vi "NI-USB6525.vi"() -> ()   [LabVIEW 2020]
doc: "test"
uses:
  LabVIEW 2020 Toolkits/toolkits_lv2020_32bit/Synchronization.llb/SynchRefs_SetGet.ctl
  LabVIEW 2020 Toolkits/VI Server Toolkit/VI Server Libraries/VI Server_GetControl.llb/VI Server_STR_Get.vi
  LabVIEW 2020 Toolkits/VI Server Toolkit/VI Server Libraries/VI Server_Set Controls.llb/Set STR Control.vi
  LabVIEW 2020 Toolkits/VI Server Toolkit/VI Server Libraries/VI Server_SetControl.llb/VI Server_BOOL_Set.vi
  LabVIEW 2020 Toolkits/VI Server Toolkit/VI Server Libraries/VI Server_SetControl.llb/VI Server_U32_Set.vi
  LabVIEW 2020 Toolkits/VI Server Toolkit/VI Server Libraries/VI Server_SetControl.llb/VI Server_1D_BOOL_Set.vi
  LabVIEW 2020 Toolkits/VI Server Toolkit/VI Server Libraries/VI Server_GetControl.llb/VI Server_DAQmx_Device_Get.vi
  LabVIEW 2020 Toolkits/VI Server Toolkit/VI Server Toolkit LV2013.lvlib
panel:
  in  "LastAction.AddToSecuence":bool
  in  "Help":bool
  in  "FP.Hide":bool caption="FrontPanel.Hide"
  out "System.Message":string caption="System Message"
  in  "EXIT":bool
  in  "Tab.Main":enum32{"Digital I/O", "Sequence", "SETTINGS"}(tab)
  in  "DataConverter.Number":u8 caption="Number"
  in  "DataConverter.Array":bool[](array[boolean])
  out "DI.Number":u8 caption="DI Number"
  out "Relay.State.Verify":bool caption="Verified"
  in  "RelayPort.Num":u8
  in  "Relay.RST":bool
  in  "RelayPort":bool[](array[boolean]) caption="Relay Port"
  out "Relay.Port.State.Verify":bool caption="Verified"
  in  "R8":bool
  in  "R7":bool
  in  "R6":bool
  in  "R5":bool
  in  "R4":bool
  in  "R3":bool
  in  "R2":bool
  in  "R1":bool
  out "DI.8":bool caption="DI 8"
  out "DI.7":bool caption="DI 7"
  out "DI.6":bool caption="DI 6"
  out "DI.5":bool caption="DI 5"
  out "DI.4":bool caption="DI 4"
  out "DI.3":bool caption="DI 3"
  out "DI.2":bool caption="DI 2"
  out "DI.1":bool caption="DI 1"
  in  "TestCase.Execute.All":bool
  in  "TestCase.Execute.Selected":bool
  out "TestCase.SAVE.Success":bool
  in  "TestCase.SAVE":bool
  in  "SequenceFile.Open":bool
  in  "SequenceFile":path caption="Secuence File"
  in  "TestCase.Execute.Step.Pause":bool
  in  "TestCase.Execute.Steps":u16(ring) caption="Test Case: Pause Before Step" items=["1", "2", "3", "4", "5", "6", "7", "8", "9", "10", "11", "12", "13", "14", "15", "16", "17", "18", "19", "20", "21", "22", "23", "24", "25", "26", "27", "28", "29", "30"]
  in  "TestCase.Execute.ABORT":bool
  in  "TestCase.Execute.Next":bool
  in  "TestCase.Execute.Pause":bool
  out "TestCase.ExecutionTime":dbl caption="Execution Time:" format="%0.3f sec"
  in  "TestCase.Execution.StepTime":u32 caption="Seq. Execution: Step Time" format="%d msec"
  in  "TestCaseConfiguration":i32[](listbox) caption="Test Case Configuration"
  in  "TestCase.StepDescription":string caption="Step Description:"
  in  "UDP.Test.String1.SendLocal":bool caption="UDP.Test.String1.Send"
  in  "ProductType":string="NI-USB6525" caption="Product Type"
  in  "VI.WindowsTitle":string="NI-USB6525" caption="Windows Title"
  in  "DAQmx.Device":tag="NI-USB6525" caption="DAQmx: Device"
  in  "Cont.Measurements.CycleTime":u32 caption="Continius Measurements:\nCycleTime"
  in  "UDP.Test.String2.Send":bool
  in  "UDP.Test.String2":string caption="UDP: Test String 2"
  in  "UDP.Port.BC":u16=58433 caption="UDP: Port.BC"
  in  "UDP.Port.RT":u16=58432 caption="UDP: Port.RT"
  in  "UDP.LocalPort":u16=58434 caption="UDP: Local Port"
  in  "UDP.IP.Address":string="234.5.6.7" caption="UDP: IP Address"
  in  "UDP.Test.String1.Send.ToInstr":bool caption="UDP.Test.String1.Send"
  in  "UDP.Test.String1":string caption="UDP: Test String 1"
  in  "UDP.Responce.String.Monitor":bool
  out "UDP.ExecEng.Message.String":string caption="UDP: Execution Engine Message String"
  out "error out":errorcluster={"status"=TRUE, "code"=1055, "source"="Property Node in VI Server Toolkit LV2013.lvlib:VI server_Set Control Value from String Format.vi:5200001->DMM6500_UDP_ExecEng_Instruction_APPLY.vi->DMM6500_UDP_MAIN.vi->Keithley2100.vi"}
  in  "error in":errorcluster
  # "15JUN2022"
  # "Digital Inputs"
  # "Data Converter"
  # "RELAYS"
  # "ON"
  # "OFF"
  # "M"
  # "Multicast IP addresses must be in the 224.0.0.0 to 239.255.255.255 range."
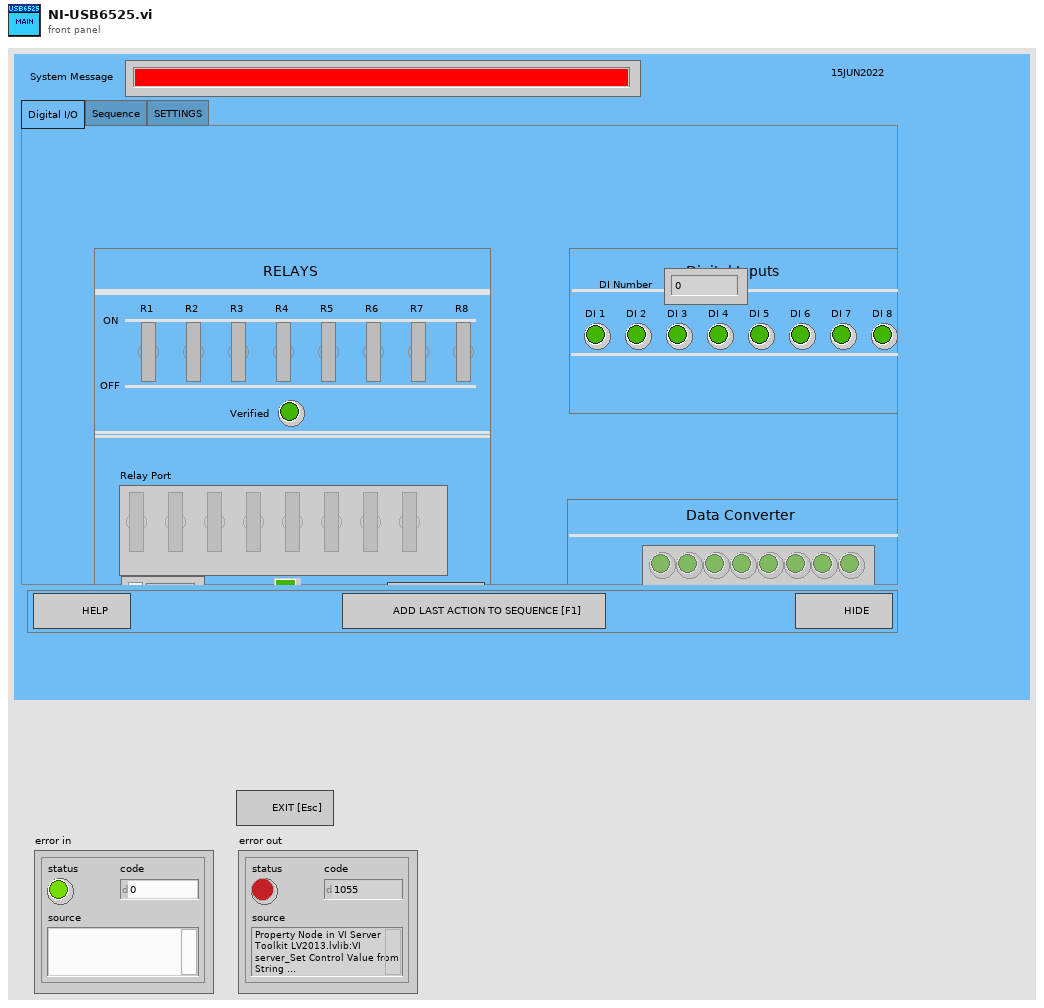
[diagram p1: front panel]
types:
  T1 = typedef "VI Server_RefsCluster.ctl" = cluster{"Labels":string[], "Refs":refnum<vi>[], "VI Ref":refnum<vi>}
  T2 = typedef "SynchRefs_SetGet.ctl" = enum16{"Set", "Get"}
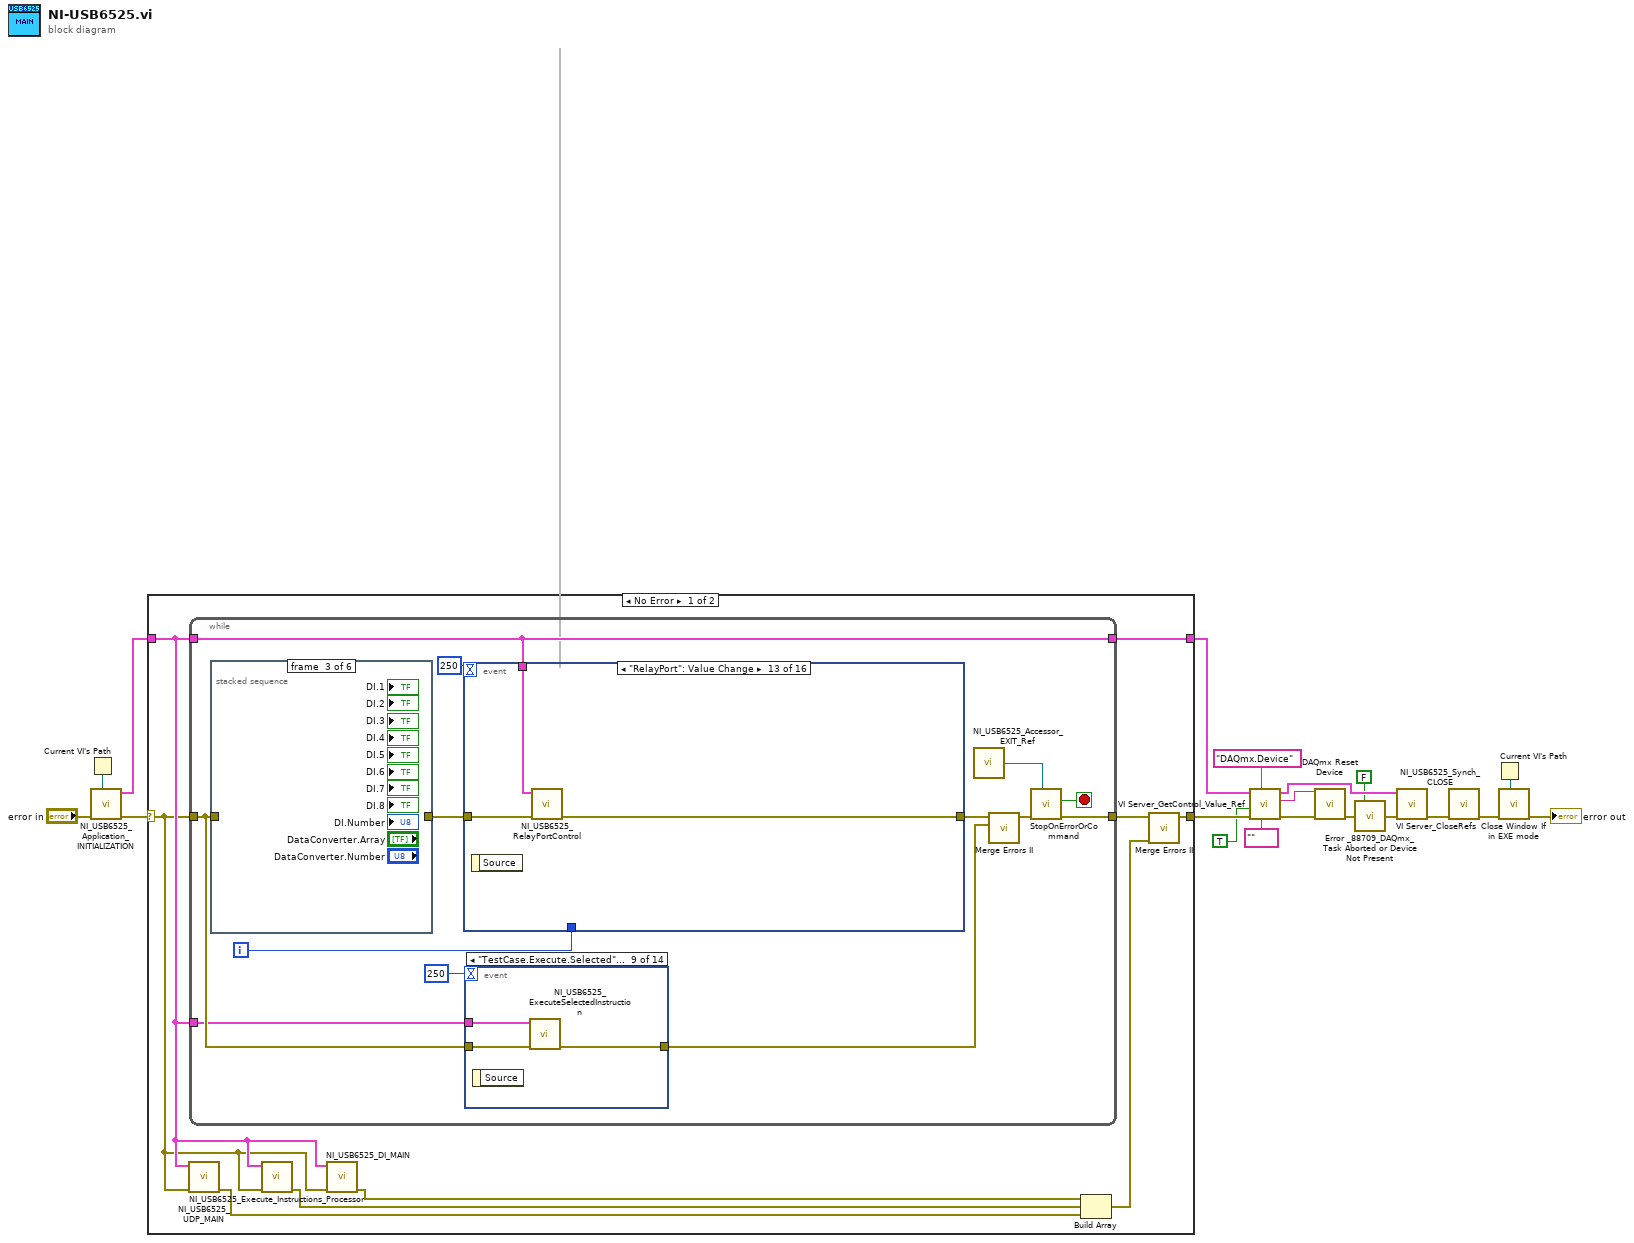
[diagram p0: block diagram]
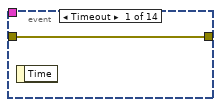
[diagram p2: hidden frame]
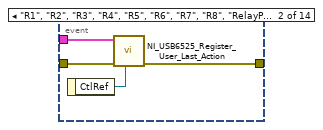
[diagram p3: hidden frame]
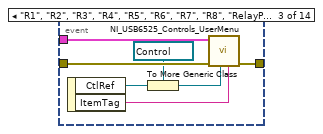
[diagram p4: hidden frame]
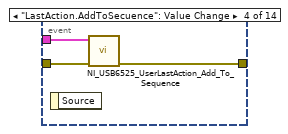
[diagram p5: hidden frame]
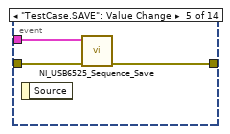
[diagram p6: hidden frame]
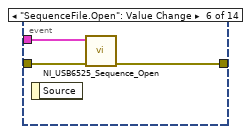
[diagram p7: hidden frame]
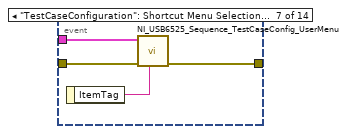
[diagram p8: hidden frame]
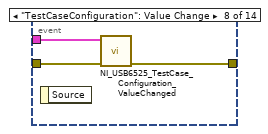
[diagram p9: hidden frame]
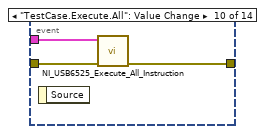
[diagram p10: hidden frame]
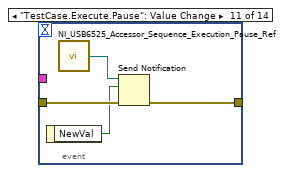
[diagram p11: hidden frame]
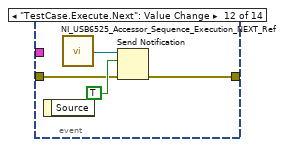
[diagram p12: hidden frame]
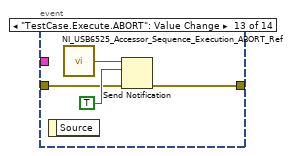
[diagram p13: hidden frame]
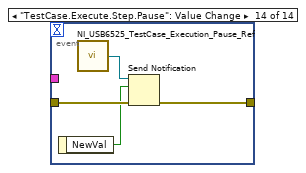
[diagram p14: hidden frame]
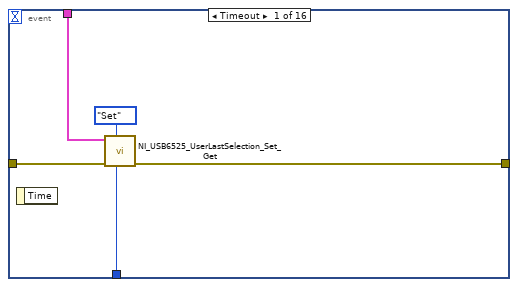
[diagram p15: hidden frame]
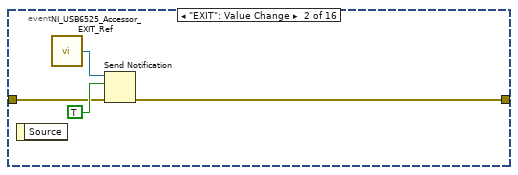
[diagram p16: hidden frame]
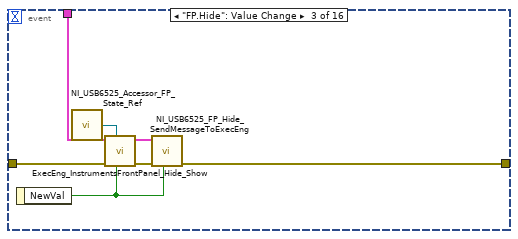
[diagram p17: hidden frame]
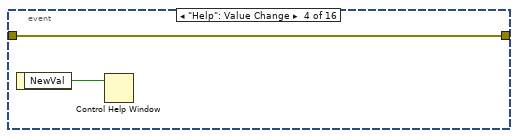
[diagram p18: hidden frame]
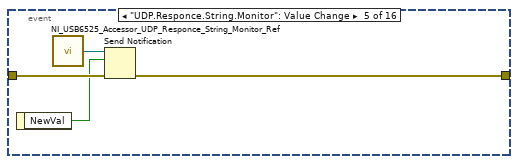
[diagram p19: hidden frame]
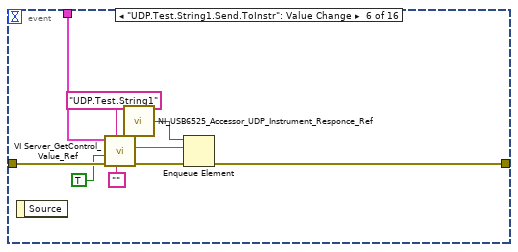
[diagram p20: hidden frame]
diagram:
  n1 = Current VI's Path() -> (path=w3:path)
  n2 = call "NI_USB6525_Application_INITIALIZATION.vi"("Top VI Path"=w3, "error in (no error)"="error in") -> ("error out"=w19:errorcluster, "VI Server Cluster.OUT"=w2:T1)  [unwired: 8 in]
  n3 = case shown="No Error" w19 {
    selector: w19 -> [w21 w192]
    tunnel: [w25 w192] -> w13
    tunnel: w2 -> [w22 w191]
    tunnel: [w28 w191] -> w11
    frame No Error {
      n4 = call "NI_USB6525_UDP_MAIN.vi"("error in (no error)"=w21, "VI Server.RefsCluster"=w22) -> ("error out"=w27:errorcluster)  [unwired: 9 in]
      n5 = while {
        tunnel: w21 -> [w33]
        tunnel: [w37] -> w26
        tunnel: w22 -> [w38]
        tunnel: [w38] -> w28
        tunnel: w22 -> [w29]
        i -> [w39]
        stop <- w36 stop-if-true
        n6 = stacked-sequence {
          tunnel: w33 -> [w190 _ _ _ _ _]
          tunnel: [w190 _ _ _ _ _] -> w41
          frame #0 {
          }
          frame #1 {
          }
          frame #2 {
          }
          frame #3 {
          }
          frame #4 {
          }
          frame #5 {
          }
        }
        n7 = event shown="[12] \"RelayPort\": Value Change" {
          selector: _ -> [_ _ _ _ _ _ _ _ _ _ _ _ _ _ _ _]
          dyn-events: _ -> [_ _ _ _ _ _ _ _ _ _ _ _ _ _ _ _]
          timeout: 250 -> [_ _ _ _ _ _ _ _ _ _ _ _ _ _ _ _]
          tunnel: w41 -> [w95 w97 w107 w109 w113 w122 w131 w140 w144 w155 w158 w168 w172 w175 w181 w188]
          tunnel: w39 -> [w94 _ _ _ _ _ _ _ _ _ _ _ _ _ _ _]
          tunnel: [w92 w99 w102 w109 w111 w120 w129 w138 w142 w153 w161 w169 w171 w173 w176 w187] -> w32
          tunnel: w38 -> [w93 _ w106 _ _ w119 w128 w137 w141 w154 w156 w166 w170 w174 w178 w186]
          event Timeout {
            n8 = event-data() -> ()  [unwired: 1 in, 1 out]
            n9 = call "NI_USB6525_UserLastSelection_Set_Get.vi"("LoopCounter"=w94, "SynchRefs.Set/Get"=SynchRefs_SetGet."Set", "error in"=w95, "VI Server.RefsCluster"=w93) -> ("error out"=w92:errorcluster)  [unwired: 6 in, 1 out]
          }
          event "EXIT": Value Change {
            n10 = event-data() -> ()  [unwired: 1 in, 1 out]
            n11 = call "NI_USB6525_Accessor_EXIT_Ref.vi"() -> ("EXIT"=w100:refnum<notifier>)  [unwired: 6 in]
            n12 = Send Notification(notification=TRUE, notifier=w100, error in (no error)=w97) -> (error out=w99:errorcluster)  [unwired: 1 out]
          }
          event "FP.Hide": Value Change {
            n13 = event-data() -> ("NewVal"=w101:bool)  [unwired: 1 in]
            n14 = call "NI_USB6525_Accessor_FP_State_Ref.vi"() -> ("FP.State"=w105:refnum<notifier>)  [unwired: 6 in]
            n15 = call "ExecEng_InstrumentsFrontPanel_Hide_Show.vi"("FP.Hide/Show"=w101, "FP.State"=w105, "error in (no error)"=w107, "VI Server Cluster"=w106) -> ("error out"=w103:errorcluster, "VI Server Cluster DUP"=w104:T1)  [unwired: 6 in]
            n16 = call "NI_USB6525_FP_Hide_SendMessageToExecEng.vi"("FP.Open"=w101, "error in (no error)"=w103, "VI Server Cluster"=w104) -> ("error out"=w102:errorcluster)  [unwired: 8 in]
          }
          event "Help": Value Change {
            n17 = event-data() -> ("NewVal"=w108:bool)  [unwired: 1 in]
            n18 = Control Help Window(1:w108) -> ()  [unwired: 1 in]
          }
          event "UDP.Responce.String.Monitor": Value Change {
            n19 = event-data() -> ("NewVal"=w110:bool)  [unwired: 1 in]
            n20 = call "NI_USB6525_Accessor_UDP_Responce_String_Monitor_Ref.vi"() -> ("UDP.ExecEng.Command.String.Monitor"=w112:refnum<notifier>)  [unwired: 6 in]
            n21 = Send Notification(notification=w110, notifier=w112, error in (no error)=w113) -> (error out=w111:errorcluster)  [unwired: 1 out]
          }
          event "UDP.Test.String1.Send.ToInstr": Value Change {
            n22 = event-data() -> ()  [unwired: 1 in, 1 out]
            n23 = call-poly "VI Server_GetControl_Value_Ref.vi"("DataType"="", "Control.Label"="UDP.Test.String1", "error in"=w122, "SingleInstance"=TRUE, "VI Server.RefsCluster"=w119) -> ("error out"=w121:errorcluster, "Value"=w114:string)  [unwired: 3 in, 2 out]
            n24 = call "NI_USB6525_Accessor_UDP_Instrument_Responce_Ref.vi"() -> ("UDP.Instrument.Responce.Q"=w115:refnum<queue>)  [unwired: 6 in]
            n25 = Enqueue Element(queue=w115, element=w114, error in (no error)=w121) -> (error out=w120:errorcluster)  [unwired: 1 in, 2 out]
          }
          event "UDP.Test.String1.SendLocal": Value Change {
            n26 = event-data() -> ()  [unwired: 1 in, 1 out]
            n27 = call-poly "VI Server_GetControl_Value_Ref.vi"("DataType"="", "Control.Label"="UDP.Test.String1", "error in"=w131, "SingleInstance"=TRUE, "VI Server.RefsCluster"=w128) -> ("error out"=w130:errorcluster, "Value"=w124:string)  [unwired: 3 in, 2 out]
            n28 = call "NI_USB6525_Accessor_UDP_ExecEng_Instruction_Q_Ref.vi"() -> ("UDP.ExecEng.Instruction.Q"=w123:refnum<queue>)  [unwired: 6 in]
            n29 = Enqueue Element(queue=w123, element=w124, error in (no error)=w130) -> (error out=w129:errorcluster)  [unwired: 1 in, 2 out]
          }
          event "UDP.Test.String2.Send": Value Change {
            n30 = event-data() -> ()  [unwired: 1 in, 1 out]
            n31 = call-poly "VI Server_GetControl_Value_Ref.vi"("DataType"="", "Control.Label"="UDP.Test.String2", "error in"=w140, "SingleInstance"=TRUE, "VI Server.RefsCluster"=w137) -> ("error out"=w139:errorcluster, "Value"=w132:string)  [unwired: 3 in, 2 out]
            n32 = call "NI_USB6525_Accessor_UDP_Instrument_Responce_Ref.vi"() -> ("UDP.Instrument.Responce.Q"=w133:refnum<queue>)  [unwired: 6 in]
            n33 = Enqueue Element(queue=w133, element=w132, error in (no error)=w139) -> (error out=w138:errorcluster)  [unwired: 1 in, 2 out]
          }
          event "UDP.ExecEng.Message.String": Shortcut Menu Selection (User) {
            n34 = event-data() -> ("ItemTag"=w143:string)  [unwired: 1 in]
            n35 = case shown="\"Clear Indicator\"" w143 {
              tunnel: w144 -> [w145 w151]
              tunnel: [w145 w150] -> w142
              tunnel: w141 -> [_ w149]
              frame "", Default {
              }
              frame "Clear Indicator" {
                n36 = call-poly "VI Server_Set Control Value.vi"("New Value"="", "Label"="UDP.ExecEng.Message.String" ("Control.Label"), "error in"=w151, "Single Instance (T)"=TRUE ("SingleInstance"), "VI Server Cluster"=w149) -> ("error out"=w150:errorcluster)  [unwired: 4 in, 2 out]
              }
            }
          }
          event "DAQmx.Device": Value Change {
            n37 = event-data() -> ("NewVal"=w152:tag)  [unwired: 1 in]
            n38 = call "NI_USB6525_DAQmx_DeviceName_Changed_UpdateSet_Get_Sections.vi"("DAQmx.Device"=w152, "error in (no error)"=w155, "VI Server Cluster"=w154) -> ("error out"=w153:errorcluster)  [unwired: 8 in]
          }
          event "Relay.RST": Value Change {
            n39 = event-data() -> ()  [unwired: 1 in, 1 out]
            n40 = call "NI_USB6525_Relays_RST.vi"("error in (no error)"=w158, "VI Server Cluster"=w156) -> ("error out"=w159:errorcluster, "VI Server Cluster.DUP"=w157:T1)  [unwired: 8 in]
            n41 = call "Time Delay"("error in (no error)"=w159, "Delay Time (s)"=0.75) -> ("error out"=w164:errorcluster)  [unwired: 9 in]
            n42 = call-poly "VI Server_SetControl.vi"("Data"=FALSE ("SingleInstance"), "Control.Label"="Relay.RST", "error in"=w164, "SingleInstance"=TRUE, "VI Server.RefsCluster"=w157) -> ("error out"=w161:errorcluster)  [unwired: 4 in, 2 out]
          }
          event "R1", "R2", "R3", "R4", "R5", "R6", "R7", "R8": Value Change {
            n43 = event-data() -> ("CtlRef"=w167:refnum<vi>)  [unwired: 1 in]
            n44 = call "NI_USB6525_RelayControl.vi"("Relay.Ref"=w167, "error in (no error)"=w168, "VI Server Cluster"=w166) -> ("error out"=w169:errorcluster)  [unwired: 8 in]
          }
          event "RelayPort": Value Change {
            n45 = event-data() -> ()  [unwired: 1 in, 1 out]
            n46 = call "NI_USB6525_RelayPortControl.vi"("error in (no error)"=w172, "VI Server Cluster"=w170) -> ("error out"=w171:errorcluster)  [unwired: 9 in]
          }
          event "RelayPort.Num": Value Change {
            n47 = event-data() -> ()  [unwired: 1 in, 1 out]
            n48 = call "NI_USB6525_RelayPortControl_Numeric.vi"("error in (no error)"=w175, "VI Server Cluster"=w174) -> ("error out"=w173:errorcluster)  [unwired: 9 in]
          }
          event "DataConverter.Array": Value Change {
            n49 = event-data() -> ("NewVal"=w182:bool[])  [unwired: 1 in]
            n50 = Boolean Array To Number(Boolean array=w182) -> (number=w179:u32)
            n51 = call-poly "VI Server_SetControl.vi"("Data"=w179, "Control.Label"="DataConverter.Number", "error in"=w181, "SingleInstance"=TRUE, "VI Server.RefsCluster"=w178) -> ("error out"=w176:errorcluster)  [unwired: 4 in, 2 out]
          }
          event "DataConverter.Number": Value Change {
            n52 = event-data() -> ("NewVal"=w189:u8)  [unwired: 1 in]
            n53 = Number To Boolean Array(number=w189) -> (Boolean array=w185:bool[])
            n54 = call-poly "VI Server_SetControl.vi"("Data"=w185, "Control.Label"="DataConverter.Array", "error in"=w188, "SingleInstance"=TRUE, "VI Server.RefsCluster"=w186) -> ("error out"=w187:errorcluster)  [unwired: 5 in, 1 out]
          }
        }
        n55 = event shown="[8] \"TestCase.Execute.Selected\": Value Change" {
          selector: _ -> [_ _ _ _ _ _ _ _ _ _ _ _ _ _]
          dyn-events: _ -> [_ _ _ _ _ _ _ _ _ _ _ _ _ _]
          timeout: 250 -> [_ _ _ _ _ _ _ _ _ _ _ _ _ _]
          tunnel: w33 -> [w42 w46 w52 w56 w59 w62 w66 w69 w72 w75 w78 w81 w85 w90]
          tunnel: [w42 w44 w51 w55 w57 w60 w63 w67 w70 w73 w77 w80 w84 w89] -> w30
          tunnel: w29 -> [_ w45 w53 w54 w58 w61 w65 w68 w71 w74 _ _ _ _]
          event Timeout {
            n56 = event-data() -> ()  [unwired: 1 in, 1 out]
          }
          event "R1", "R2", "R3", "R4", "R5", "R6", "R7", "R8", "RelayPort", "Relay.RST", "RelayPort.Num": Value Change {
            n57 = event-data() -> ("CtlRef"=w43:refnum<vi>)  [unwired: 1 in]
            n58 = call "NI_USB6525_Register_User_Last_Action.vi"("CtlRef"=w43, "error in (no error)"=w46, "VI Server Cluster"=w45) -> ("error out"=w44:errorcluster)  [unwired: 7 in, 1 out]
          }
          event "R1", "R2", "R3", "R4", "R5", "R6", "R7", "R8", "RelayPort.Num", "Relay.RST", "RelayPort": Shortcut Menu Selection (User) {
            n59 = event-data() -> ("CtlRef"=w48:refnum<vi>, "ItemTag"=w50:string)  [unwired: 1 in]
            n60 = To More Generic Class(target class=refnum<vi> refnum ("Control Reference (Generic)"), reference=w48) -> (generic class reference=w47:refnum<vi>)
            n61 = call "NI_USB6525_Controls_UserMenu.vi"("ItemTag"=w50, "Control Ref"=w47, "error in (no error)"=w52, "VI Server Cluster"=w53) -> ("error out"=w51:errorcluster)  [unwired: 7 in]
          }
          event "LastAction.AddToSecuence": Value Change {
            n62 = event-data() -> ()  [unwired: 1 in, 1 out]
            n63 = call "NI_USB6525_UserLastAction_Add_To_Sequence.vi"("error in (no error)"=w56, "VI Server Cluster"=w54) -> ("error out"=w55:errorcluster)  [unwired: 9 in]
          }
          event "TestCase.SAVE": Value Change {
            n64 = event-data() -> ()  [unwired: 1 in, 1 out]
            n65 = call "NI_USB6525_Sequence_Save.vi"("error in (no error)"=w59, "VI Server Cluster"=w58) -> ("error out"=w57:errorcluster)  [unwired: 9 in]
          }
          event "SequenceFile.Open": Value Change {
            n66 = event-data() -> ()  [unwired: 1 in, 1 out]
            n67 = call "NI_USB6525_Sequence_Open.vi"("error in (no error)"=w62, "VI Server Cluster"=w61) -> ("error out"=w60:errorcluster)  [unwired: 9 in]
          }
          event "TestCaseConfiguration": Shortcut Menu Selection (User) {
            n68 = event-data() -> ("ItemTag"=w64:string)  [unwired: 1 in]
            n69 = call "NI_USB6525_Sequence_TestCaseConfig_UserMenu.vi"("ItemTag"=w64, "error in (no error)"=w66, "VI Server.RefsCluster"=w65) -> ("error out"=w63:errorcluster)  [unwired: 8 in]
          }
          event "TestCaseConfiguration": Value Change {
            n70 = event-data() -> ()  [unwired: 1 in, 1 out]
            n71 = call "NI_USB6525_TestCase_Configuration_ValueChanged.vi"("error in"=w69, "VI Server.RefsCluster"=w68) -> ("error out"=w67:errorcluster)  [unwired: 8 in, 1 out]
          }
          event "TestCase.Execute.Selected": Value Change {
            n72 = event-data() -> ()  [unwired: 1 in, 1 out]
            n73 = call "NI_USB6525_ExecuteSelectedInstruction.vi"("error in (no error)"=w72, "VI Server Cluster"=w71) -> ("error out"=w70:errorcluster)  [unwired: 9 in]
          }
          event "TestCase.Execute.All": Value Change {
            n74 = event-data() -> ()  [unwired: 1 in, 1 out]
            n75 = call "NI_USB6525_Execute_All_Instruction.vi"("error in (no error)"=w75, "VI Server Cluster"=w74) -> ("error out"=w73:errorcluster)  [unwired: 9 in]
          }
          event "TestCase.Execute.Pause": Value Change {
            n76 = event-data() -> ("NewVal"=w76:bool)  [unwired: 1 in]
            n77 = call "NI_USB6525_Accessor_Sequence_Execution_Pause_Ref.vi"() -> ("SequenceExecution.PAUSE"=w79:refnum<notifier>)  [unwired: 6 in]
            n78 = Send Notification(notification=w76, notifier=w79, error in (no error)=w78) -> (error out=w77:errorcluster)  [unwired: 1 out]
          }
          event "TestCase.Execute.Next": Value Change {
            n79 = event-data() -> ()  [unwired: 1 in, 1 out]
            n80 = call "NI_USB6525_Accessor_Sequence_Execution_NEXT_Ref.vi"() -> ("SequenceExecution.NEXT"=w83:refnum<notifier>)  [unwired: 6 in]
            n81 = Send Notification(notification=TRUE, notifier=w83, error in (no error)=w81) -> (error out=w80:errorcluster)  [unwired: 1 out]
          }
          event "TestCase.Execute.ABORT": Value Change {
            n82 = event-data() -> ()  [unwired: 1 in, 1 out]
            n83 = call "NI_USB6525_Accessor_Sequence_Execution_ABORT_Ref.vi"() -> ("SequenceExecution.ABORT"=w86:refnum<notifier>)  [unwired: 6 in]
            n84 = Send Notification(notification=TRUE, notifier=w86, error in (no error)=w85) -> (error out=w84:errorcluster)  [unwired: 1 out]
          }
          event "TestCase.Execute.Step.Pause": Value Change {
            n85 = event-data() -> ("NewVal"=w88:bool)  [unwired: 1 in]
            n86 = call "NI_USB6525_TestCase_Execution_Pause_Ref.vi"() -> ("SequenceExecution.StepPAUSE"=w91:refnum<notifier>)  [unwired: 6 in]
            n87 = Send Notification(notification=w88, notifier=w91, error in (no error)=w90) -> (error out=w89:errorcluster)  [unwired: 1 out]
          }
        }
        n88 = call "NI_USB6525_Accessor_EXIT_Ref.vi"() -> ("EXIT"=w35:refnum<notifier>)  [unwired: 6 in]
        n89 = call "Merge Errors II.vi"("error in 2 (no error)"=w30, "error in 1 (no error)"=w32) -> ("error out.DUP"=w31:errorcluster)  [unwired: 4 in, 1 out]
        n90 = call "StopOnErrorOrCommand.vi"("STOP"=w35, "error in (no error)"=w31) -> ("error out"=w37:errorcluster, "STOP"=w36:bool)  [unwired: 8 in]
      }
      n91 = call "NI_USB6525_Execute_Instructions_Processor.vi"("error in (no error)"=w21, "VI Server.RefsCluster"=w22) -> ("error out"=w23:errorcluster)  [unwired: 9 in]
      n92 = call "NI_USB6525_DI_MAIN.vi"("error in (no error)"=w21, "VI Server Cluster"=w22) -> ("error out"=w20:errorcluster)  [unwired: 9 in]
      n93 = Build Array(w20, w23, w27) -> (w24:errorcluster[])
      n94 = call "Merge Errors II.vi"("error array in"=w24, "error in 1 (no error)"=w26) -> ("error out.DUP"=w25:errorcluster)  [unwired: 4 in, 1 out]
    }
    frame Error {
    }
  }
  n95 = call-poly "VI Server_GetControl_Value_Ref.vi"("DataType"=tag "" ("DAQmx.Device"), "Control.Label"="DAQmx.Device", "error in"=w13, "SingleInstance"=TRUE, "VI Server.RefsCluster"=w11) -> ("error out"=w16:errorcluster, "Value"=w17:tag, "VI Server.RefsCluster.DUP"=w12:T1)  [unwired: 3 in, 1 out]
  n96 = call <vilib>:"DAQmx Reset Device.vi"("device in"=w17, "error in"=w16) -> ("error out"=w6:errorcluster)  [unwired: 13 in]
  n97 = call "Error _88709_DAQmx_Task Aborted or Device Not Present.vi"("Display Error Message"=FALSE, "error in"=w6) -> ("error out"=w5:errorcluster)  [unwired: 12 in, 1 out]
  n98 = call "VI Server_CloseRefs.vi"("error in"=w5, "VI Server.RefsCluster"=w12) -> ("error out"=w18:errorcluster)  [unwired: 9 in]
  n99 = call "NI_USB6525_Synch_CLOSE.vi"("error in"=w18) -> ("error out"=w9:errorcluster)  [unwired: 10 in]
  n100 = Current VI's Path() -> (path=w7:path)
  n101 = call "Close Window If in EXE mode.vi"("TopLevelVI Path"=w7, "error in"=w9) -> ("error out"=→"error out":errorcluster)  [unwired: 9 in]
